vi "Initialize IMU.vi"(8 "error in (no error)":errorcluster, 11 "IMU VISA":refnum<visa-resource-name>="COM5") -> (0 "error out":errorcluster, 3 "VISA resource name out":refnum<visa-resource-name>)   [LabVIEW 2012]
uses:
  <vilib>/Instr/_visa.llb/VISA Configure Serial Port (Instr).vi
  IMU/LabVIEW Library v2/AHRS/SubVI/3DM-GX3-45 Commands/Start Stream.vi
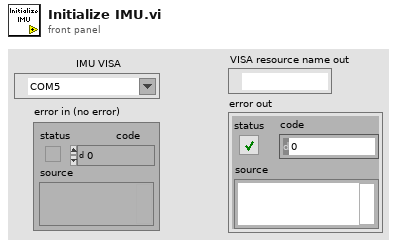
[diagram p1: front panel]
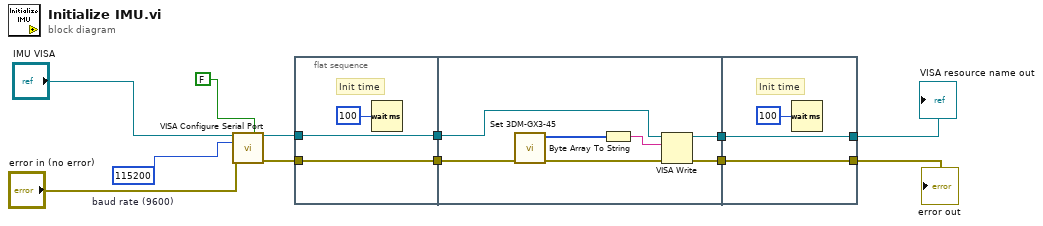
[diagram p0: block diagram]
diagram:
  w7 = u32 115200  # baud rate (9600)
  n1 = call-poly "VISA Configure Serial Port"("VISA resource name"="IMU VISA", "Enable Termination\nChar (T)"=FALSE ("Enable Termination\nChar (T)"), "baud rate (9600)"=w7, "error in (no error)"="error in (no error)") -> ("VISA resource name out"=w5:refnum<visa-resource-name>, "error out"=w4:errorcluster)  [unwired: 10 in]
  n2 = flat-sequence {
    tunnel: w5 -> [w15]
    tunnel: w4 -> [w13]
    tunnel: [w15] -> w12
    tunnel: [w13] -> w11
    tunnel: w12 -> [w19]
    tunnel: w11 -> [w18]
    tunnel: [w17] -> w10
    tunnel: [w16] -> w9
    tunnel: [w24] -> w2
    tunnel: [w25] -> w3
    tunnel: w10 -> [w25]
    tunnel: w9 -> [w24]
    frame #0 {
      # "Init time"
      n3 = Wait (ms)(milliseconds to wait=u32 100) -> ()  [unwired: 1 out]
    }
    frame #1 {
      n4 = call-poly "Set 3DM-GX3-45.vi"("Error In"=w18) -> ("Error Out"=w22:errorcluster, "Command"=w20:u8[])  [unwired: 9 in]
      n5 = Byte Array To String(unsigned byte array=w20) -> (string=w21:string)
      n6 = VISA Write(VISA resource name=w19, write buffer=w21, error in (no error)=w22) -> (VISA resource name out=w16:refnum<visa-resource-name>, error out=w17:errorcluster)  [unwired: 1 out]
    }
    frame #2 {
      # "Init time"
      n7 = Wait (ms)(milliseconds to wait=u32 100) -> ()  [unwired: 1 out]
    }
  }
  "VISA resource name out" <- w2
  "error out" <- w3
